vi "VisionExecute.v.vi"   [LabVIEW 2023]
uses:
  <vilib>/Rock Robotics/WPI/ThirdParty/PhotonVisionLib/Enum/PhotonPoseStrategy_ENUM.ctl
  <vilib>/Rock Robotics/WPI/ThirdParty/JAS_Junk/TrajLib/TypeDef/POSE2D.ctl
  <vilib>/Rock Robotics/WPI/ThirdParty/JAS_Junk/TrajLib/TypeDef/TRANSLATION2D.ctl
  <vilib>/Rock Robotics/WPI/ThirdParty/JAS_Junk/TrajLib/TypeDef/ROTATION2D.ctl
  <vilib>/Rock Robotics/WPI/ThirdParty/JAS_Junk/TrajLib/VI/AprilTagFieldLayout_New2025.vi
  <vilib>/Rock Robotics/WPI/ThirdParty/JAS_Junk/TrajLib/VI/Util_GetTime_U32.vi
  <vilib>/Rock Robotics/WPI/ThirdParty/PhotonVisionLib/SubVI/PhotonPipelineResult_Unpack.vi
  <vilib>/Rock Robotics/WPI/ThirdParty/PhotonVisionLib/SubVI/PhotonPipelineResult_GetTargetCount.vi
  <vilib>/Rock Robotics/WPI/ThirdParty/PhotonVisionLib/SubVI/PhotonPipelineResult_GetMetadata.vi
  <vilib>/Rock Robotics/WPI/ThirdParty/PhotonVisionLib/SubVI/PhotonPipelineMetadata_GetAll.vi
  <vilib>/Rock Robotics/WPI/ThirdParty/JAS_Junk/TrajLib/VI/Transform3d_Equals.vi
  <vilib>/Rock Robotics/WPI/ThirdParty/PhotonVisionLib/SubVI/PhotonPoseEstimator_SetCamera.vi
  <vilib>/Rock Robotics/WPI/ThirdParty/PhotonVisionLib/SubVI/PhotonPoseEstimator_SetPrimaryStategy.vi
  <vilib>/Rock Robotics/WPI/ThirdParty/PhotonVisionLib/SubVI/PhotonPoseEstimator_SetMultiTagFallbackStrategy.vi
  <vilib>/Rock Robotics/WPI/ThirdParty/PhotonVisionLib/SubVI/PhotonPoseEstimator_SetHighestAmbiguity.vi
  <vilib>/Rock Robotics/WPI/ThirdParty/PhotonVisionLib/SubVI/PhotonPoseEstimator_SetRobotToCameraTransform.vi
  <vilib>/Rock Robotics/WPI/ThirdParty/PhotonVisionLib/SubVI/PhotonPoseEstimator_New.vi
  <vilib>/Rock Robotics/WPI/ThirdParty/PhotonVisionLib/SubVI/PhotonPoseEstimator_SetLastPose.vi
  <vilib>/Rock Robotics/WPI/ThirdParty/PhotonVisionLib/SubVI/PhotonPoseEstimator_Update_PipeResult.vi
  <vilib>/Rock Robotics/WPI/ThirdParty/PhotonVisionLib/SubVI/PhotonPoseEstimator_SetReferencePose.vi
  <vilib>/Rock Robotics/WPI/ThirdParty/PhotonVisionLib/SubVI/PhotonEstimatedRobotPose_GetAll.vi
  <vilib>/Rock Robotics/WPI/ThirdParty/JAS_Junk/TrajLib/VI/Pose3d_ToPose2d.vi
  <vilib>/Rock Robotics/WPI/ThirdParty/JAS_Junk/TrajLib/VI/Quaternion_New.vi
  <vilib>/Rock Robotics/WPI/ThirdParty/JAS_Junk/TrajLib/Conv_Deg_Radians.vi
  <vilib>/Rock Robotics/WPI/ThirdParty/JAS_Junk/TrajLib/Translation2d_GetDistance.vi
  <vilib>/Rock Robotics/WPI/ThirdParty/JAS_Junk/TrajLib/Rotation2d_Minus.vi
  <vilib>/Rock Robotics/WPI/ThirdParty/JAS_Junk/TrajLib/Rotation2d_GetRadians.vi
  <vilib>/Rock Robotics/WPI/ThirdParty/JAS_Junk/TrajLib/VI/AprilTagFieldLayout_New.vi
  <vilib>/Rock Robotics/WPI/ThirdParty/JAS_Junk/TrajLib/VI/Pose3d_New_Trans3dRot3d.vi
  <vilib>/Rock Robotics/WPI/ThirdParty/JAS_Junk/TrajLib/VI/Rotation3d_Create_Quaternion.vi
  <vilib>/Rock Robotics/WPI/ThirdParty/JAS_Junk/TrajLib/VI/AprilTag_New.vi
  <vilib>/Rock Robotics/WPI/ThirdParty/JAS_Junk/TrajLib/Timer_New.vi
  <vilib>/Rock Robotics/WPI/ThirdParty/PhotonVisionLib/SubVI/Packet_decode_ByteI8.vi
  <vilib>/Rock Robotics/WPI/ThirdParty/PhotonVisionLib/SubVI/PhotonTrackedTarget_Unpack.vi
  <vilib>/Rock Robotics/WPI/ThirdParty/PhotonVisionLib/SubVI/PhotonMultiTargetPNPResult_unpack.vi
  <vilib>/Rock Robotics/WPI/ThirdParty/PhotonVisionLib/SubVI/PhotonPipelineMetadata_Unpack.vi
  <vilib>/Rock Robotics/WPI/ThirdParty/PhotonVisionLib/SubVI/PhotonPipelineResult_New.vi
  <vilib>/Rock Robotics/WPI/ThirdParty/JAS_Junk/TrajLib/VI/Transform3d_GetTranslation3d.vi
  <vilib>/Rock Robotics/WPI/ThirdParty/JAS_Junk/TrajLib/VI/Transform3d_GetRotation3d.vi
  <vilib>/Rock Robotics/WPI/ThirdParty/JAS_Junk/TrajLib/VI/Rotation3d_Equals.vi
  <vilib>/Rock Robotics/WPI/ThirdParty/JAS_Junk/TrajLib/VI/Translation3d_Equals.vi
  <vilib>/Rock Robotics/WPI/ThirdParty/PhotonVisionLib/SubVI/PhotonTargetModel_New_AprilTag36H11.vi
  <vilib>/Rock Robotics/WPI/ThirdParty/PhotonVisionLib/SubVI/PhotonPoseEstimator_Update_All.vi
  <vilib>/Rock Robotics/WPI/ThirdParty/JAS_Junk/TrajLib/VI/Pose3d_getTranslation3d.vi
  <vilib>/Rock Robotics/WPI/ThirdParty/JAS_Junk/TrajLib/VI/Pose3d_getRotation3d.vi
  <vilib>/Rock Robotics/WPI/ThirdParty/JAS_Junk/TrajLib/VI/Translation3d_ToTranslation2d.vi
  <vilib>/Rock Robotics/WPI/ThirdParty/JAS_Junk/TrajLib/VI/Rotation3d_ToRotation2d.vi
  <vilib>/Rock Robotics/WPI/ThirdParty/JAS_Junk/TrajLib/Pose2d_New_TRRO.vi
  <vilib>/Rock Robotics/WPI/ThirdParty/JAS_Junk/TrajLib/Util_CalcDist.vi
  <vilib>/Rock Robotics/WPI/ThirdParty/JAS_Junk/TrajLib/Rotation2d_UnaryMinus.vi
  <vilib>/Rock Robotics/WPI/ThirdParty/JAS_Junk/TrajLib/Rotation2d_RotateBy.vi
  <vilib>/Rock Robotics/WPI/ThirdParty/JAS_Junk/TrajLib/VI/AprilTag_GetAll.vi
  <vilib>/Rock Robotics/WPI/ThirdParty/JAS_Junk/TrajLib/VI/Quaternion_Normalize.vi
  <vilib>/Rock Robotics/WPI/ThirdParty/PhotonVisionLib/SubVI/Packet_decode_Flt64.vi
  <vilib>/Rock Robotics/WPI/ThirdParty/PhotonVisionLib/SubVI/TargetCorner_New.vi
  <vilib>/Rock Robotics/WPI/ThirdParty/PhotonVisionLib/SubVI/Packet_decode_Int32.vi
  <vilib>/Rock Robotics/WPI/ThirdParty/PhotonVisionLib/SubVI/Packet_decode_Transform3d.vi
  <vilib>/Rock Robotics/WPI/ThirdParty/PhotonVisionLib/SubVI/Packet_decode_Flt32.vi
  <vilib>/Rock Robotics/WPI/ThirdParty/PhotonVisionLib/SubVI/Packet_decode_TargetCornerArray.vi
  <vilib>/Rock Robotics/WPI/ThirdParty/PhotonVisionLib/SubVI/Packet_decode_Boolean.vi
  <vilib>/Rock Robotics/WPI/ThirdParty/PhotonVisionLib/SubVI/PhotonPNPResult_unpack.vi
  <vilib>/Rock Robotics/WPI/ThirdParty/PhotonVisionLib/SubVI/PhotonMultiTargetPNPResult_New.vi
  <vilib>/Rock Robotics/WPI/ThirdParty/PhotonVisionLib/SubVI/Packet_decode_Int16.vi
  <vilib>/Rock Robotics/WPI/ThirdParty/PhotonVisionLib/SubVI/Packet_decode_Int64.vi
  <vilib>/Rock Robotics/WPI/ThirdParty/JAS_Junk/TrajLib/VI/Rotation3d_GetQuaterion.vi
  <vilib>/Rock Robotics/WPI/ThirdParty/JAS_Junk/TrajLib/VI/Quaternion_Equals.vi
  <vilib>/Rock Robotics/WPI/ThirdParty/PhotonVisionLib/SubVI/PhotonTargetModel_New_RectPlanar.vi
  <vilib>/Rock Robotics/WPI/ThirdParty/PhotonVisionLib/SubVI/PhotonPoseEstimator_GetEmptyPose.vi
  <vilib>/Rock Robotics/WPI/ThirdParty/PhotonVisionLib/SubVI/PhotonPoseEstimator_lowestAmbiguityStrategy.vi
  <vilib>/Rock Robotics/WPI/ThirdParty/PhotonVisionLib/SubVI/PhotonPoseEstimator_closestToCameraHeightStrategy.vi
  <vilib>/Rock Robotics/WPI/ThirdParty/PhotonVisionLib/SubVI/PhotonPoseEstimator_closestToReferencePoseStrategy.vi
  <vilib>/Rock Robotics/WPI/ThirdParty/PhotonVisionLib/SubVI/PhotonPoseEstimator_GetReferencePose.vi
  <vilib>/Rock Robotics/WPI/ThirdParty/PhotonVisionLib/SubVI/PhotonPoseEstimator_GetLastPose.vi
  <vilib>/Rock Robotics/WPI/ThirdParty/PhotonVisionLib/SubVI/PhotonPoseEstimator_averageBestTargetsStrategy.vi
  <vilib>/Rock Robotics/WPI/ThirdParty/PhotonVisionLib/SubVI/PhotonPoseEstimator_multiTagOnCoprocStrategy.vi
  <vilib>/Rock Robotics/WPI/ThirdParty/PhotonVisionLib/SubVI/PhotonPipelineResult_GetTimeStampSecs.vi
  <vilib>/Rock Robotics/WPI/ThirdParty/JAS_Junk/TrajLib/Translation2d_Create.vi
  <vilib>/Rock Robotics/WPI/ThirdParty/JAS_Junk/TrajLib/Rotation2d_CreateAngle.vi
  <vilib>/Rock Robotics/WPI/ThirdParty/JAS_Junk/TrajLib/VI/Rotation3d_GetXYZ.vi
  <vilib>/Rock Robotics/WPI/ThirdParty/JAS_Junk/TrajLib/Rotation2d_CreateXY.vi
  <vilib>/Rock Robotics/WPI/ThirdParty/JAS_Junk/TrajLib/VI/Quaternion_New_Default.vi
  <vilib>/Rock Robotics/WPI/ThirdParty/PhotonVisionLib/SubVI/PhotonPNPResult_New.vi
  <vilib>/Rock Robotics/WPI/ThirdParty/JAS_Junk/TrajLib/VI/Quaternion_Get_Vect.vi
  <vilib>/Rock Robotics/WPI/ThirdParty/JAS_Junk/TrajLib/VI/Quaternion_Get_W.vi
  <vilib>/Rock Robotics/WPI/ThirdParty/PhotonVisionLib/SubVI/PhotonTargetModel_New.vi
  <vilib>/Rock Robotics/WPI/ThirdParty/JAS_Junk/TrajLib/VI/Rotation3d_Create_AxisAngle.vi
  <vilib>/Rock Robotics/WPI/ThirdParty/JAS_Junk/TrajLib/VI/Pose3d_New.vi
  <vilib>/Rock Robotics/WPI/ThirdParty/PhotonVisionLib/SubVI/PhotonPipelineResult_HasTargets.vi
  <vilib>/Rock Robotics/WPI/ThirdParty/PhotonVisionLib/SubVI/PhotonPipelineResult_GetTargets.vi
  <vilib>/Rock Robotics/WPI/ThirdParty/PhotonVisionLib/SubVI/PhotonTrackedTarget_GetPoseAmbiguity.vi
  <vilib>/Rock Robotics/WPI/ThirdParty/PhotonVisionLib/SubVI/PhotonTrackedTarget_GetFiducialId.vi
  <vilib>/Rock Robotics/WPI/ThirdParty/PhotonVisionLib/SubVI/PhotonPoseEstimator_GetFieldTags.vi
  <vilib>/Rock Robotics/WPI/ThirdParty/JAS_Junk/TrajLib/VI/AprilTagFieldLayout_GetTagPose.vi
  <vilib>/Rock Robotics/WPI/ThirdParty/JAS_Junk/TrajLib/VI/Pose3d_TransformBy.vi
  <vilib>/Rock Robotics/WPI/ThirdParty/PhotonVisionLib/SubVI/PhotonTrackedTarget_GetBestCameraToTarget.vi
  <vilib>/Rock Robotics/WPI/ThirdParty/JAS_Junk/TrajLib/VI/Transform3d_Inverse.vi
  <vilib>/Rock Robotics/WPI/ThirdParty/PhotonVisionLib/SubVI/PhotonPoseEstimator_GetRobotToCameraTransform.vi
  <vilib>/Rock Robotics/WPI/ThirdParty/PhotonVisionLib/SubVI/PhotonPoseEstimator_GetHighestAmbiguity.vi
  <vilib>/Rock Robotics/WPI/ThirdParty/PhotonVisionLib/SubVI/PhotonEstimatedRobotPose_New.vi
  <vilib>/Rock Robotics/WPI/ThirdParty/PhotonVisionLib/SubVI/PhotonPoseEstimator_closestToCameraHeightStrategy_calc.vi
  <vilib>/Rock Robotics/WPI/ThirdParty/PhotonVisionLib/SubVI/PhotonTrackedTarget_GetAltCameraToTarget.vi
  <vilib>/Rock Robotics/WPI/ThirdParty/PhotonVisionLib/SubVI/PhotonPoseEstimator_closestToReferencePoseStrategy_calc.vi
  <vilib>/Rock Robotics/WPI/ThirdParty/PhotonVisionLib/SubVI/PhotonPoseEstimator_averageBestTargetsStrategy_calc.vi
  <vilib>/Rock Robotics/WPI/ThirdParty/JAS_Junk/TrajLib/VI/Rotation3d_Plus.vi
  <vilib>/Rock Robotics/WPI/ThirdParty/JAS_Junk/TrajLib/VI/Translation3d_Plus.vi
  <vilib>/Rock Robotics/WPI/ThirdParty/JAS_Junk/TrajLib/VI/Translation3d_Times.vi
  <vilib>/Rock Robotics/WPI/ThirdParty/JAS_Junk/TrajLib/VI/Rotation3d_Times.vi
  <vilib>/Rock Robotics/WPI/ThirdParty/JAS_Junk/TrajLib/VI/Rotation3d_Create_Default.vi
  <vilib>/Rock Robotics/WPI/ThirdParty/JAS_Junk/TrajLib/VI/Translation3d_Create_Default.vi
  <vilib>/Rock Robotics/WPI/ThirdParty/JAS_Junk/TrajLib/VI/Pose3d_New_Default.vi
  <vilib>/Rock Robotics/WPI/ThirdParty/JAS_Junk/TrajLib/VI/Pose3d_Plus.vi
  <vilib>/Rock Robotics/WPI/ThirdParty/JAS_Junk/TrajLib/VI/Pose3d_RelativeTo.vi
  <vilib>/Rock Robotics/WPI/ThirdParty/JAS_Junk/TrajLib/VI/AprilTagFieldLayout_GetOriginPosition.vi
  <vilib>/Rock Robotics/WPI/ThirdParty/PhotonVisionLib/SubVI/PhotonPipelineResult_GetMultiTagResult.vi
  <vilib>/Rock Robotics/WPI/ThirdParty/JAS_Junk/TrajLib/VI/Quaternion_Get_All.vi
  <vilib>/Rock Robotics/WPI/ThirdParty/JAS_Junk/TrajLib/VI/Vector_Norm.vi
  <vilib>/Rock Robotics/WPI/ThirdParty/JAS_Junk/TrajLib/VecBuilder_ArrayBy1Fill.vi
  <vilib>/Rock Robotics/WPI/ThirdParty/JAS_Junk/TrajLib/VI/Translation3d_RotateBy.vi
  <vilib>/Rock Robotics/WPI/ThirdParty/JAS_Junk/TrajLib/Transform2d_Create_TransRot.vi
  <vilib>/Rock Robotics/WPI/ThirdParty/JAS_Junk/TrajLib/VI/Rotation3d_UnaryMinus.vi
  <vilib>/Rock Robotics/WPI/ThirdParty/JAS_Junk/TrajLib/VI/Translation3d_UnaryMinus.vi
  <vilib>/Rock Robotics/WPI/ThirdParty/JAS_Junk/TrajLib/VI/Transform3d_GetXYZ.vi
  <vilib>/Rock Robotics/WPI/ThirdParty/JAS_Junk/TrajLib/VI/Pose3d_getXYZ.vi
  <vilib>/Rock Robotics/WPI/ThirdParty/PhotonVisionLib/SubVI/PhotonPoseEstimator_CalcDifference.vi
  <vilib>/Rock Robotics/WPI/ThirdParty/JAS_Junk/TrajLib/VI/Rotation3d_RotateBy.vi
  <vilib>/Rock Robotics/WPI/ThirdParty/JAS_Junk/TrajLib/VI/Translation3d_GetXYZ.vi
  <vilib>/Rock Robotics/WPI/ThirdParty/JAS_Junk/TrajLib/VI/Transform3d_Create_Pose3dPose3d.vi
  <vilib>/Rock Robotics/WPI/ThirdParty/JAS_Junk/TrajLib/MatBuilder_Create.vi
  <vilib>/Rock Robotics/WPI/ThirdParty/JAS_Junk/TrajLib/VI/Quaternion_Times.vi
  <vilib>/Rock Robotics/WPI/ThirdParty/JAS_Junk/TrajLib/VI/Quaternion_Inverse.vi
  <vilib>/Rock Robotics/WPI/ThirdParty/JAS_Junk/TrajLib/VI/Translation3d_GetDistance.vi
  <vilib>/Rock Robotics/WPI/ThirdParty/JAS_Junk/TrajLib/VI/Translation3d_Minus.vi
  <vilib>/Rock Robotics/WPI/ThirdParty/JAS_Junk/TrajLib/VI/Rotation3d_Minus.vi
  Robot Global Data.vi
  VisionGlobal.vi
  <vilib>/Rock Robotics/SystemInterfaces/Utilities/FPGA_UtilitiesRead LocalTime.vi
  <vilib>/Rock Robotics/WPI/ThirdParty/JAS_Junk/TrajLib/VI/Util_GetTime_U64.vi
  <vilib>/Utility/semaphor.llb/Obtain Semaphore Reference.vi
  <vilib>/Rock Robotics/WPI/ThirdParty/JAS_Junk/TrajLib/Timer_Reset.vi
  <vilib>/Rock Robotics/WPI/ThirdParty/JAS_Junk/TrajLib/Timer_Start.vi
  <vilib>/Rock Robotics/WPI/ThirdParty/JAS_Junk/TrajLib/Timer_Stop.vi
  <vilib>/Rock Robotics/WPI/ThirdParty/JAS_Junk/TrajLib/Timer_HasPeriodPassedOnce.vi
  <vilib>/Rock Robotics/Network Tables/NT Read Value.vi
  <vilib>/Rock Robotics/Network Tables/NT Read Raw.vi
  <vilib>/Rock Robotics/WPI/ThirdParty/JAS_Junk/TrajLib/Trajectory_Library.lvlib
  <vilib>/Rock Robotics/WPI/ThirdParty/PhotonVisionLib/PhotonVisionLib.lvlib
types:
  T1 = typedef "PhotonVisionLib.lvlib/PhotonPoseStrategy_ENUM.ctl" = enum16{"LOWEST_AMBIGUITY", "CLOSEST_TO_CAMERA_HEIGHT", "CLOSEST_TO_REFERENCE_POSE", "CLOSEST_TO_LAST_POSE", "AVERAGE_BEST_TARGETS", "MULTI_TAG_PNP_ON_COPROCESSOR", "MULTI_TAG_PNP_ON_RIO"}
  T2 = typedef "Trajectory_Library.lvlib/TRANSLATION3D.ctl" = cluster{"X":dbl, "Y":dbl, "Z":dbl}
  T3 = typedef "Trajectory_Library.lvlib/ROTATION3D.ctl" = cluster{"Q_quaternion":T4}
  T4 = typedef "Trajectory_Library.lvlib/QUATERNION.ctl" = cluster{"R":dbl, "V":dbl[]}
  T5 = typedef "Trajectory_Library.lvlib/TRANSFORM3D.ctl" = cluster{"TRANSLATION3D":T2, "ROTATION3D":T3, "XF":bool}
  T6 = typedef "PhotonVisionLib.lvlib/PhotonPipelineResultType.ctl" = cluster{"Targets":T7[], "PhotonMultiTargetPNPResult":T9, "PhotonPipelineMetadata":T11}
  T7 = typedef "PhotonVisionLib.lvlib/PhotonTrackedTargetType.ctl" = cluster{"Yaw":dbl, "Pitch":dbl, "Area":dbl, "Skew":dbl, "MinAreaRectCorners":T8[], "BestCameraToTarget":T5, "FiducialId":i32, "AltCameraToTarget":T5, "PoseAmbiguity":dbl, "DetectedCorners":T8[], "ObjDetectId":i32, "ObjDetectConf":sgl}
  T8 = typedef "PhotonVisionLib.lvlib/TargetCornerType.ctl" = cluster{"X":dbl, "Y":dbl}
  T9 = typedef "PhotonVisionLib.lvlib/PhotonMultiTargetPNPResultType.ctl" = cluster{"PhotonPNPResult":T10, "FiducialIDsUsed":i16[]}
  T10 = typedef "PhotonVisionLib.lvlib/PhotonPNPResultType.ctl" = cluster{"IsPresent":bool, "bestReprojErr":dbl, "altReprojErr":dbl, "ambiguity":dbl, "Best":T5, "Alt":T5}
  T11 = typedef "PhotonVisionLib.lvlib/PhotonPipelineMetadataType.ctl" = cluster{"CaptureTimestampMicros":i64, "PublishTimestampMicros":i64, "SequenceID":i64, "TimeSinceLastPong":i64}
  T12 = typedef "Trajectory_Library.lvlib/AprilTagFieldLayout.ctl" = cluster{"AprilTagMap":map{i32, T13}, "FieldLength":dbl, "FieldWidth":dbl, "OriginPosition ":T15, "OriginPose3d":T14}
  T13 = typedef "Trajectory_Library.lvlib/AprilTag.ctl" = cluster{"ID":i32, "POSE3D":T14}
  T14 = typedef "Trajectory_Library.lvlib/POSE3D.ctl" = cluster{"Translation3d":T2, "Rotation3d":T3}
  T15 = typedef "Trajectory_Library.lvlib/AprilTagFieldLayoutOrignPosition_ENUM.ctl" = enum16{"kBlueAllianceWallRightSide,", "kRedAllianceWallRightSide,"}
  T16 = typedef "PhotonVisionLib.lvlib/PhotonPoseEstimator_Configuration.ctl" = cluster{"Primary Strategy":T1, "Camera":string, "Initial Pose":T14, "HighestAmbiguity":dbl, "RobotToCamera":T5, "FallBack Strategy":T1, "BaseNTName":string}
  T17 = typedef "Trajectory_Library.lvlib/SWERVE_DRIVE_KINEMATICS.ctl" = cluster{"NumModules":i32, "InverseKinematics":T18, "ForwardKinematics":T18, "Modules":T19[], "PrevCoR":T19, "SavedModuleStates":T20[]}
  T18 = typedef "NI_Matrix.lvlib/RealMatrix.ctl" = dbl[][]
  T19 = typedef "Trajectory_Library.lvlib/TRANSLATION2D.ctl" = cluster{"X":dbl, "Y":dbl}
  T20 = typedef "Trajectory_Library.lvlib/SWERVE_DRIVE_MODULE_STATE.ctl" = cluster{"Speed":dbl, "Angle":T21}
  T21 = typedef "Trajectory_Library.lvlib/ROTATION2D.ctl" = cluster{"VALUE":dbl, "COS":dbl, "SIN":dbl}
  T22 = typedef "Trajectory_Library.lvlib/SWERVE_DRIVE_MODULE_POSITION.ctl" = cluster{"Distance":dbl, "Angle":T21, "P":bool}
  T23 = typedef "Trajectory_Library.lvlib/SWERVE_DRIVE_POSE_EST2_CONFIG.ctl" = cluster{"Wheel_Locations M":T19[], "Odom X std dev M":dbl, "Odom Y std dev M":dbl, "Odom Heading std dev Rad":dbl, "Vision X std dev M":dbl, "Vision Y std dev M":dbl, "Vision Heading std dev Rad":dbl}
  T24 = typedef "Trajectory_Library.lvlib/POSE2D.ctl" = cluster{"TRANSLATION":T19, "ROTATION":T21}
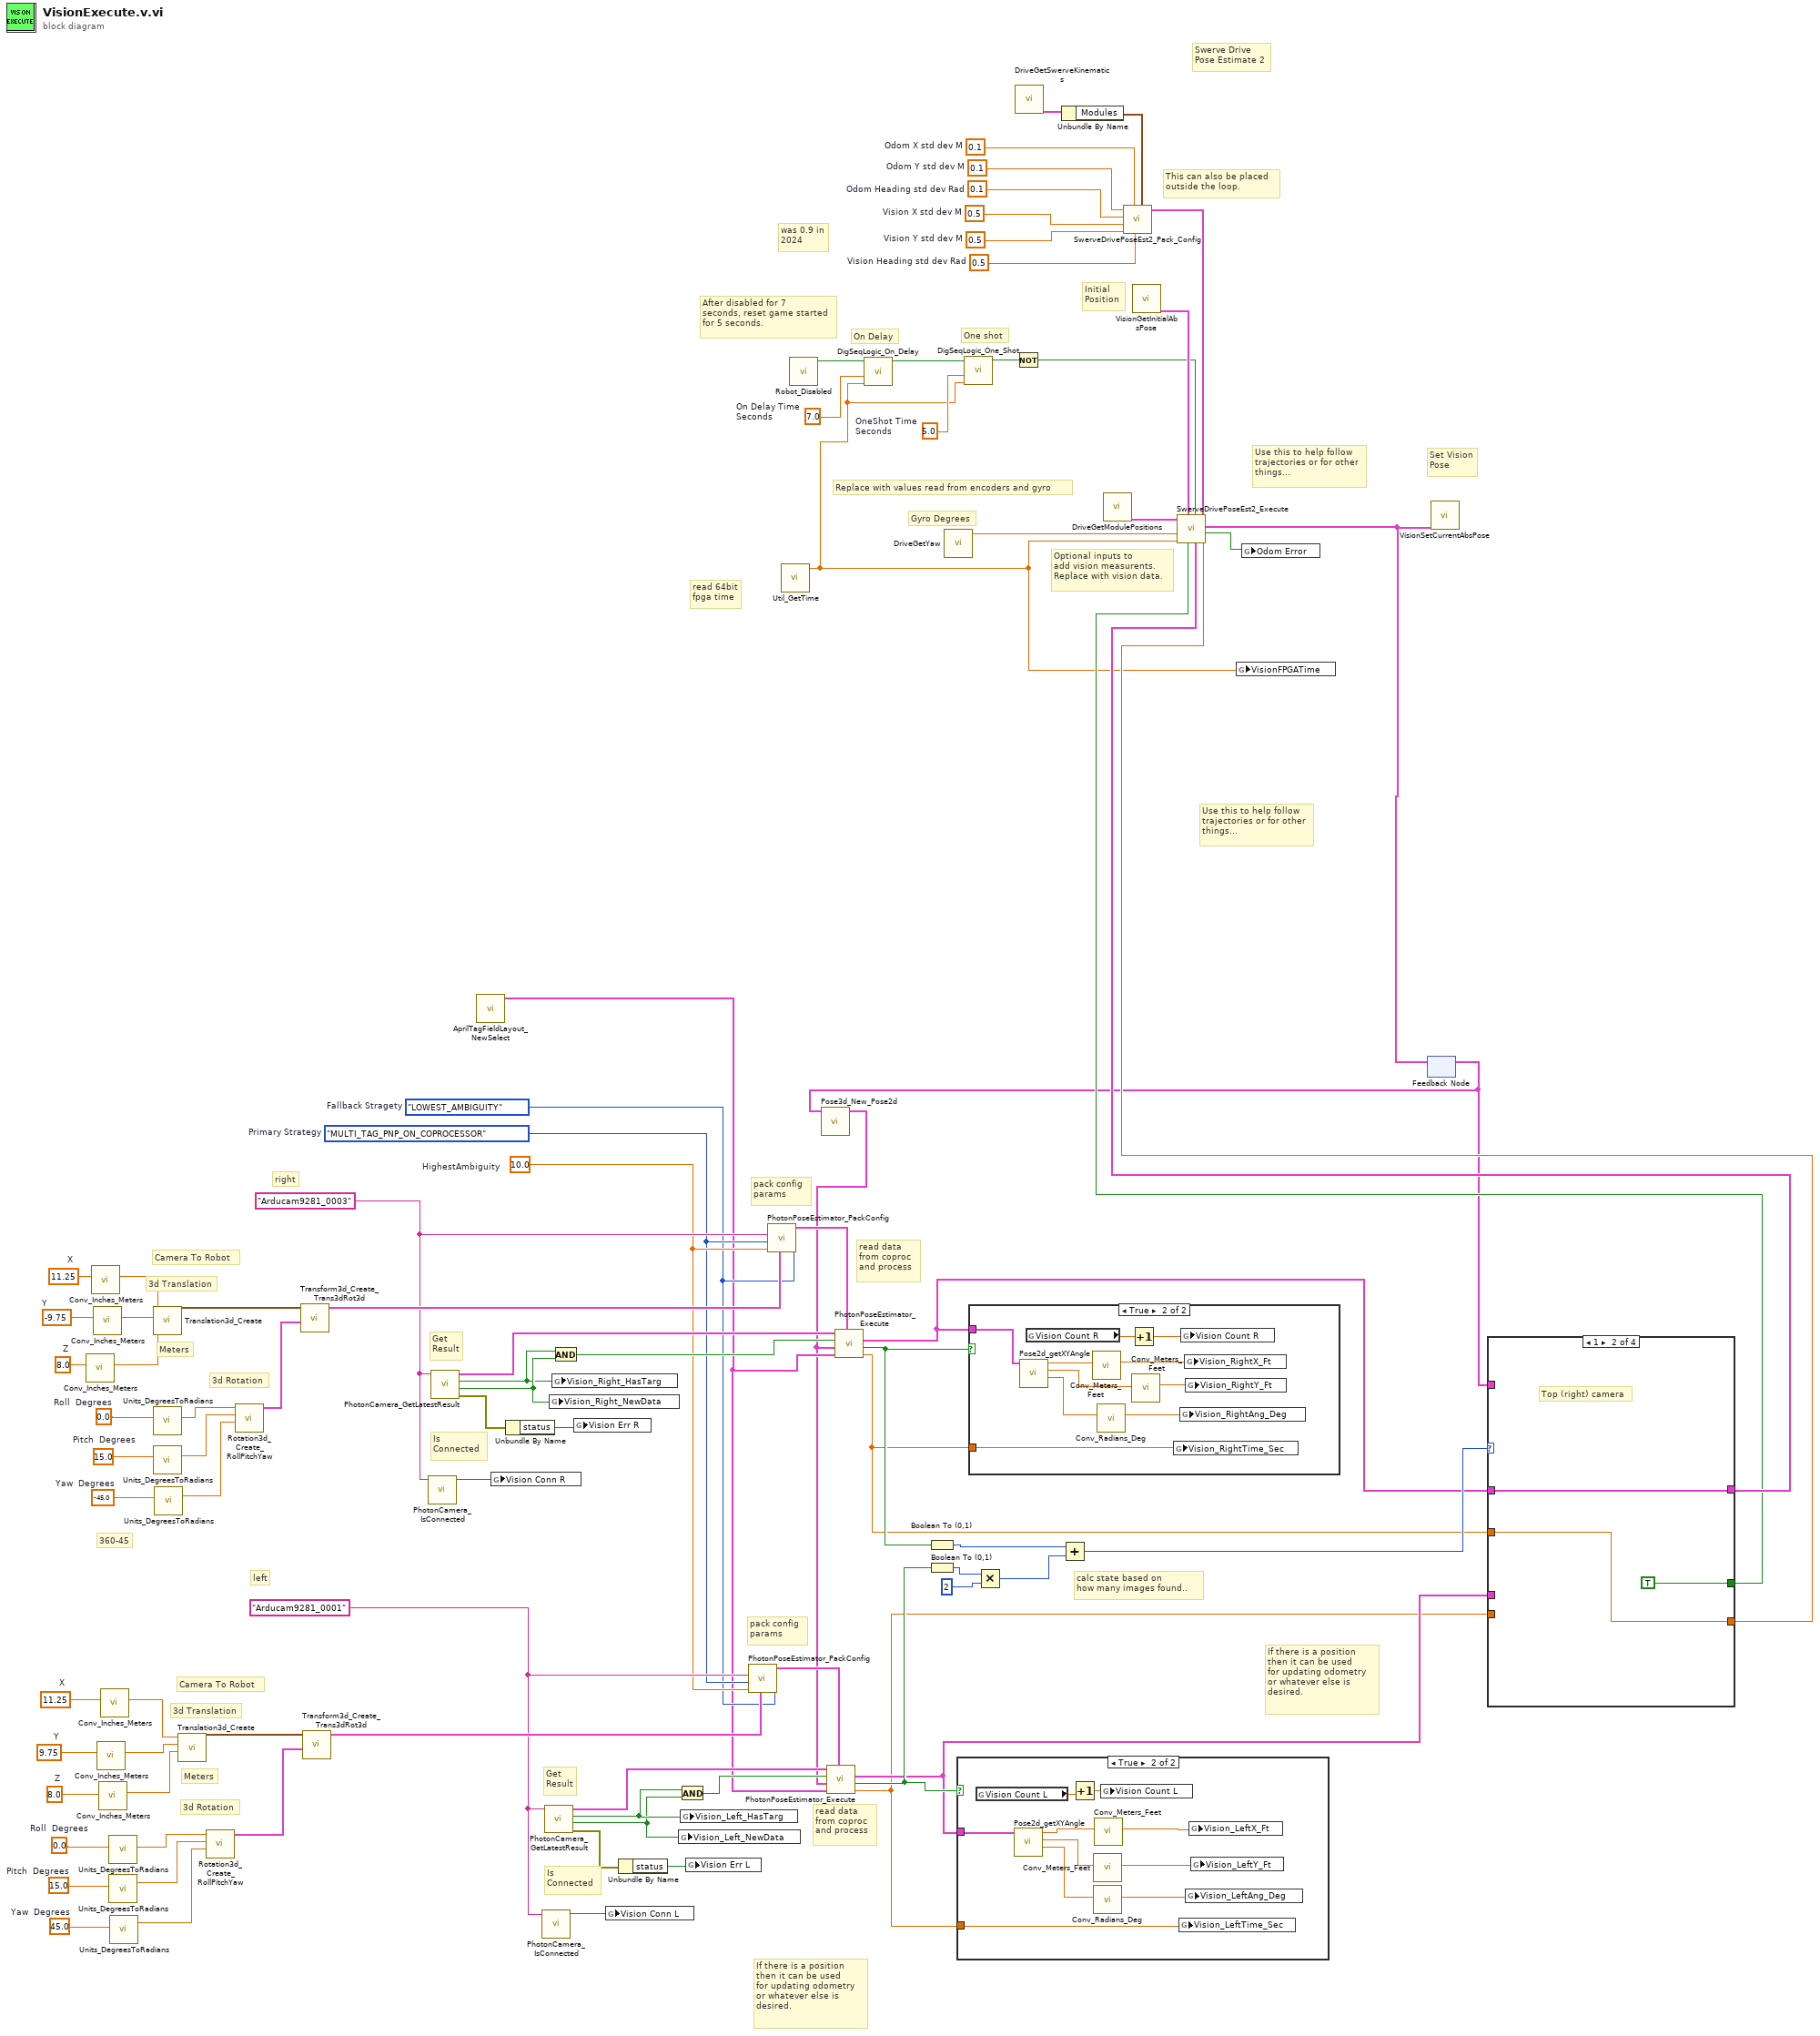
[diagram p0: block diagram]
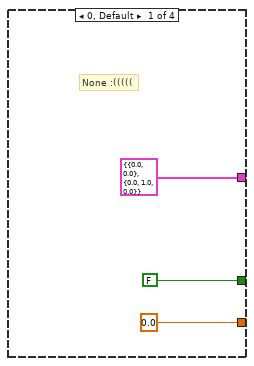
[diagram p2: hidden frame]
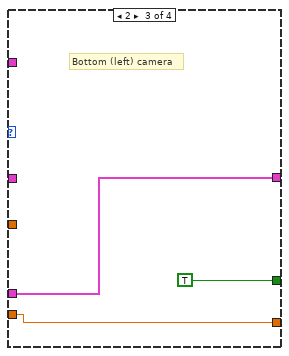
[diagram p3: hidden frame]
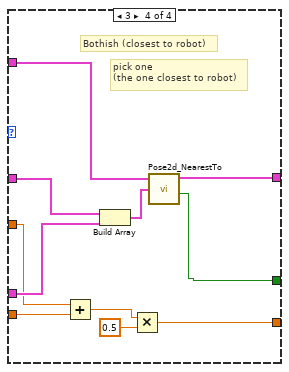
[diagram p4: hidden frame]
diagram:
  w11 = 5.0  # OneShot Time Seconds
  w13 = 7.0  # On Delay Time Seconds
  w21 = PhotonPoseStrategy_ENUM."LOWEST_AMBIGUITY"  # Fallback Stragety
  w31 = 0.1  # Odom Y std dev M
  w32 = 0.1  # Odom Heading std dev Rad
  w33 = 0.5  # Vision X std dev M
  w34 = 0.5  # Vision Y std dev M
  w35 = 0.1  # Odom X std dev M
  w36 = 0.5  # Vision Heading std dev Rad
  w68 = 0.0  # Roll  Degrees
  w67 = 15.0  # Pitch  Degrees
  w66 = 45.0  # Yaw  Degrees
  w53 = 8.0  # Z
  w57 = 11.25  # X
  w55 = 9.75  # Y
  w62 = "Arducam9281_0001" ("CameraName")
  w84 = 0.0  # Roll  Degrees
  w83 = 15.0  # Pitch  Degrees
  w82 = -45.0  # Yaw  Degrees
  w47 = 8.0  # Z
  w51 = 11.25  # X
  w49 = -9.75  # Y
  w45 = 10.0  # HighestAmbiguity
  w44 = PhotonPoseStrategy_ENUM."MULTI_TAG_PNP_ON_COPROCESSOR"  # Primary Strategy
  w78 = "Arducam9281_0003" ("CameraName")
  # "Set Vision\nPose"
  # "After disabled for 7\nseconds, reset game started\nfor 5 seconds."
  # "One shot"
  # "On Delay"
  # "360-45"
  # "was 0.9 in\n2024"
  # "calc state based on\nhow many images found.."
  # "read data\nfrom coproc\nand process"
  # "read data\nfrom coproc\nand process"
  # "pack config\nparams"
  # "pack config\nparams"
  # "Initial\nPosition"
  # "Optional inputs to\nadd vision measurents.\nReplace with vision data."
  # "Replace with values read from encoders and gyro"
  # "read 64bit\nfpga time"
  # "This can also be placed \noutside the loop."
  # "Use this to help follow\ntrajectories or for other\nthings..."
  # "Swerve Drive \nPose Estimate 2"
  # "Use this to help follow\ntrajectories or for other\nthings..."
  # "right"
  # "left"
  # "If there is a position\nthen it can be used\nfor updating odometry\nor whatever else is \ndesired."
  # "Meters"
  # "Camera To Robot"
  # "3d Rotation"
  # "3d Translation"
  # "Is\nConnected"
  # "Get\nResult"
  # "If there is a position\nthen it can be used\nfor updating odometry\nor whatever else is \ndesired."
  # "Meters"
  # "Camera To Robot"
  # "3d Rotation"
  # "3d Translation"
  # "Is\nConnected"
  # "Get\nResult"
  # "Gyro Degrees"
  n1 = call <vilib>:"Conv_Inches_Meters.vi"("INCH"=w47) -> ("Meters"=w46:dbl)  [unwired: 10 in]
  n2 = call <vilib>:"Conv_Inches_Meters.vi"("INCH"=w51) -> ("Meters"=w50:dbl)  [unwired: 10 in]
  n3 = call <vilib>:"Conv_Inches_Meters.vi"("INCH"=w49) -> ("Meters"=w48:dbl)  [unwired: 10 in]
  n4 = call <vilib>:"Conv_Inches_Meters.vi"("INCH"=w55) -> ("Meters"=w54:dbl)  [unwired: 10 in]
  n5 = call <vilib>:"Conv_Inches_Meters.vi"("INCH"=w53) -> ("Meters"=w52:dbl)  [unwired: 10 in]
  n6 = call <vilib>:"Conv_Inches_Meters.vi"("INCH"=w57) -> ("Meters"=w56:dbl)  [unwired: 10 in]
  n7 = call <vilib>:"Units_DegreesToRadians.vi"("Degrees"=w68) -> ("Radians"=w65:dbl)  [unwired: 10 in]
  n8 = call <vilib>:"Units_DegreesToRadians.vi"("Degrees"=w67) -> ("Radians"=w64:dbl)  [unwired: 10 in]
  n9 = call <vilib>:"Units_DegreesToRadians.vi"("Degrees"=w66) -> ("Radians"=w63:dbl)  [unwired: 10 in]
  n10 = call <vilib>:"Translation3d_Create.vi"("Z"=w46, "Y"=w48, "X"=w50) -> ("TRANSLATION3D"=w85:T2)  [unwired: 8 in]
  n11 = call <vilib>:"Units_DegreesToRadians.vi"("Degrees"=w84) -> ("Radians"=w81:dbl)  [unwired: 10 in]
  n12 = call <vilib>:"Units_DegreesToRadians.vi"("Degrees"=w83) -> ("Radians"=w80:dbl)  [unwired: 10 in]
  n13 = call <vilib>:"Units_DegreesToRadians.vi"("Degrees"=w82) -> ("Radians"=w79:dbl)  [unwired: 10 in]
  n14 = call <vilib>:"Translation3d_Create.vi"("Z"=w52, "Y"=w54, "X"=w56) -> ("TRANSLATION3D"=w69:T2)  [unwired: 8 in]
  n15 = call <vilib>:"Rotation3d_Create_RollPitchYaw.vi"("Yaw"=w63, "Pitch"=w64, "Roll"=w65) -> ("Rotation3d"=w70:T3)  [unwired: 8 in]
  n16 = call <vilib>:"Rotation3d_Create_RollPitchYaw.vi"("Yaw"=w79, "Pitch"=w80, "Roll"=w81) -> ("Rotation3d"=w86:T3)  [unwired: 8 in]
  n17 = call <vilib>:"Transform3d_Create_Trans3dRot3d.vi"("Rotation3d"=w86, "Translation3d"=w85) -> ("Transform3d"=w87:T5)  [unwired: 9 in]
  n18 = call <vilib>:"Transform3d_Create_Trans3dRot3d.vi"("Rotation3d"=w70, "Translation3d"=w69) -> ("Transform3d"=w71:T5)  [unwired: 9 in]
  n19 = call <vilib>:"PhotonCamera_IsConnected.vi"("CameraName"=w78) -> ("IsConnected"=w76:bool)  [unwired: 9 in, 1 out]
  n20 = call <vilib>:"PhotonCamera_GetLatestResult.vi"("CameraName"=w78) -> ("error out"=w75:errorcluster, "New Data"=w4:bool, "HasTargets"=w3:bool, "PipelineResult"=w88:T6)  [unwired: 6 in, 1 out]
  n21 = call-poly <vilib>:"AprilTagFieldLayout_NewSelect.vi"() -> ("AprilTagFieldLayout"=w14:T12)  [unwired: 11 in]
  n22 = global write "VisionGlobal.vi" "Vision Conn R"(w76) -> ()
  n23 = Unbundle By Name(w75) -> ("status"=w74:bool)
  n24 = call <vilib>:"PhotonCamera_IsConnected.vi"("CameraName"=w62) -> ("IsConnected"=w60:bool)  [unwired: 9 in, 1 out]
  n25 = call <vilib>:"PhotonCamera_GetLatestResult.vi"("CameraName"=w62) -> ("error out"=w59:errorcluster, "New Data"=w1:bool, "HasTargets"=w2:bool, "PipelineResult"=w72:T6)  [unwired: 6 in, 1 out]
  n26 = global write "VisionGlobal.vi" "Vision_Right_NewData"(w4) -> ()
  n27 = And(x=w3, y=w4) -> (x .and. y?=w89:bool)
  n28 = global write "VisionGlobal.vi" "Vision_Right_HasTarg"(w3) -> ()
  n29 = global write "VisionGlobal.vi" "Vision Err R"(w74) -> ()
  n30 = global write "VisionGlobal.vi" "Vision Conn L"(w60) -> ()
  n31 = Unbundle By Name(w59) -> ("status"=w58:bool)
  n32 = And(x=w2, y=w1) -> (x .and. y?=w73:bool)
  n33 = global write "VisionGlobal.vi" "Vision_Left_NewData"(w1) -> ()
  n34 = global write "VisionGlobal.vi" "Vision_Left_HasTarg"(w2) -> ()
  n35 = global write "VisionGlobal.vi" "Vision Err L"(w58) -> ()
  n36 = call <vilib>:"PhotonPoseEstimator_PackConfig.vi"("FallBack Strategy"=w21, "RobotToCamera"=w71, "HighestAmbiguity"=w45, "PirmaryStrategy"=w44, "Camera"=w62) -> ("PoseEstimator_Configuration"=w61:T16)  [unwired: 6 in]
  n37 = call <vilib>:"PhotonPoseEstimator_PackConfig.vi"("FallBack Strategy"=w21, "RobotToCamera"=w87, "HighestAmbiguity"=w45, "PirmaryStrategy"=w44, "Camera"=w78) -> ("PoseEstimator_Configuration"=w77:T16)  [unwired: 6 in]
  n38 = call <vilib>:"Util_GetTime.vi"() -> ("FPGA_Time_Seconds"=w7:dbl)  [unwired: 9 in, 2 out]
  n39 = call "Robot_Disabled.vi"() -> ("Robot Disabled"=w12:bool)  [unwired: 11 in]
  n40 = call <vilib>:"DigSeqLogic_On_Delay.vi"("Time"=w7, "Delay"=w13, "Input"=w12) -> ("Output"=w10:bool)  [unwired: 7 in, 1 out]
  n41 = call "DriveGetYaw.vi"() -> ("Yaw"=w26:dbl)  [unwired: 11 in]
  n42 = call <vilib>:"DigSeqLogic_One_Shot.vi"("Time"=w7, "OneShot"=w11, "Input"=w10) -> ("Output"=w9:bool)  [unwired: 7 in, 1 out]
  n43 = Not(x=w9) -> (.not. x?=w8:bool)
  n44 = call "DriveGetSwerveKinematics.vi"() -> ("SWERVE_DRIVE_KINEMATICS"=w23:T17)  [unwired: 11 in]
  n45 = Unbundle By Name(w23) -> ("Modules"=w22:T19[])
  n46 = call "DriveGetModulePositions.vi"() -> ("Swerve_Drive_Modual_Positions"=w27:T22[])  [unwired: 11 in]
  n47 = call <vilib>:"SwerveDrivePoseEst2_Pack_Config.vi"("Wheel_Locations M"=w22, "Vision Heading std dev Rad"=w36, "Odom X std dev M"=w35, "Vision Y std dev M"=w34, "Vision X std dev M"=w33, "Odom Heading std dev Rad"=w32, "Odom Y std dev M"=w31) -> ("SwervePoseEst2Config"=w30:T23)  [unwired: 4 in]
  n48 = call "VisionGetInitialAbsPose.vi"() -> ("InitialABSPose"=w15:T24)  [unwired: 10 in]
  n49 = global write "VisionGlobal.vi" "VisionFPGATime"(w7) -> ()
  n50 = feedback #1() -> (w6:T24)  [unwired: 1 in]
  n51 = call <vilib>:"Pose3d_New_Pose2d.vi"("in POSE2D"=w6) -> ("out Pose3d"=w5:T14)  [unwired: 10 in]
  n52 = call <vilib>:"PhotonPoseEstimator_Execute.vi"("Configuration"=w61, "AprilTagFieldLayout"=w14, "ReferencePose"=w5, "PIpeline Has \nNew Results"=w73, "PipelineResult"=w72) -> ("TimeStamp_Seconds"=w18:dbl, "New Pose Found"=w42:bool, "EstimatedPose2d"=w20:T24)  [unwired: 4 out]
  n53 = call <vilib>:"PhotonPoseEstimator_Execute.vi"("Configuration"=w77, "AprilTagFieldLayout"=w14, "ReferencePose"=w5, "PIpeline Has \nNew Results"=w89, "PipelineResult"=w88) -> ("TimeStamp_Seconds"=w17:dbl, "New Pose Found"=w43:bool, "EstimatedPose2d"=w19:T24)  [unwired: 4 out]
  n54 = Boolean To (0,1)(Boolean=w43) -> (0, 1=w38:i16)
  n55 = Boolean To (0,1)(Boolean=w42) -> (0, 1=w41:i16)
  n56 = case shown="True" w42 {
    tunnel: w20 -> [_ w97]
    tunnel: w18 -> [_ w90]
    frame False {
    }
    frame True {
      n57 = global read "VisionGlobal.vi" "Vision Count L"() -> (w98:dbl)
      n58 = call <vilib>:"Pose2d_getXYAngle.vi"("in POSE"=w97) -> ("Angle"=w94:dbl, "Y"=w95:dbl, "X"=w96:dbl)  [unwired: 8 in]
      n59 = Increment(x=w98) -> (x+1=w99:dbl)
      n60 = call <vilib>:"Conv_Meters_Feet.vi"("Meters"=w95) -> ("Feet"=w92:dbl)  [unwired: 10 in]
      n61 = call <vilib>:"Conv_Radians_Deg.vi"("Radians"=w94) -> ("Degrees"=w91:dbl)  [unwired: 10 in]
      n62 = call <vilib>:"Conv_Meters_Feet.vi"("Meters"=w96) -> ("Feet"=w93:dbl)  [unwired: 10 in]
      n63 = global write "VisionGlobal.vi" "Vision Count L"(w99) -> ()
      n64 = global write "VisionGlobal.vi" "Vision_LeftTime_Sec"(w90) -> ()
      n65 = global write "VisionGlobal.vi" "Vision_LeftAng_Deg"(w91) -> ()
      n66 = global write "VisionGlobal.vi" "Vision_LeftX_Ft"(w93) -> ()
      n67 = global write "VisionGlobal.vi" "Vision_LeftY_Ft"(w92) -> ()
    }
  }
  n68 = case shown="True" w43 {
    tunnel: w19 -> [_ w107]
    tunnel: w17 -> [_ w100]
    frame False {
    }
    frame True {
      n69 = call <vilib>:"Pose2d_getXYAngle.vi"("in POSE"=w107) -> ("Angle"=w104:dbl, "Y"=w105:dbl, "X"=w106:dbl)  [unwired: 8 in]
      n70 = global read "VisionGlobal.vi" "Vision Count R"() -> (w108:dbl)
      n71 = call <vilib>:"Conv_Meters_Feet.vi"("Meters"=w106) -> ("Feet"=w103:dbl)  [unwired: 10 in]
      n72 = call <vilib>:"Conv_Radians_Deg.vi"("Radians"=w104) -> ("Degrees"=w101:dbl)  [unwired: 10 in]
      n73 = Increment(x=w108) -> (x+1=w109:dbl)
      n74 = call <vilib>:"Conv_Meters_Feet.vi"("Meters"=w105) -> ("Feet"=w102:dbl)  [unwired: 10 in]
      n75 = global write "VisionGlobal.vi" "Vision_RightTime_Sec"(w100) -> ()
      n76 = global write "VisionGlobal.vi" "Vision_RightAng_Deg"(w101) -> ()
      n77 = global write "VisionGlobal.vi" "Vision Count R"(w109) -> ()
      n78 = global write "VisionGlobal.vi" "Vision_RightX_Ft"(w103) -> ()
      n79 = global write "VisionGlobal.vi" "Vision_RightY_Ft"(w102) -> ()
    }
  }
  n80 = Multiply(x=w41, y=i16 2) -> (x*y=w39:i16)
  n81 = Add(x=w38, y=w39) -> (x+y=w37:i16)
  n82 = case shown="1" w37 {
    tunnel: w19 -> [_ w114 _ w127]
    tunnel: w20 -> [_ _ w117 w126]
    tunnel: w6 -> [_ _ _ w128]
    tunnel: [FALSE ("Found") TRUE ("Found") TRUE ("Found") w124] -> w16
    tunnel: w17 -> [_ w115 _ w123]
    tunnel: w18 -> [_ _ w118 w122]
    tunnel: [T24 {"TRANSLATION"={"X"=0.0, "Y"=0.0}, "ROTATION"={"VALUE"=0.0, "COS"=1.0, "SIN"=0.0}} ("Nearest Pose") w114 w117 w125] -> w25
    tunnel: [0.0 w115 w118 w119] -> w24
    frame 0, Default {
      # "None :((((("
    }
    frame 1 {
      # "Top (right) camera"
    }
    frame 2 {
      # "Bottom (left) camera"
    }
    frame 3 {
      # "pick one \n(the one closest to robot)"
      # "Bothish (closest to robot)"
      n83 = Add(x=w123, y=w122) -> (x+y=w121:dbl)
      n84 = Build Array(w127, w126) -> (w129:T24[])
      n85 = Multiply(x=w121, y=0.5) -> (x*y=w119:dbl)
      n86 = call <vilib>:"Pose2d_NearestTo.vi"("other POSE"=w129, "in POSE"=w128) -> ("Found"=w124:bool, "Nearest Pose"=w125:T24)  [unwired: 8 in]
    }
  }
  n87 = call <vilib>:"SwerveDrivePoseEst2_Execute.vi"("Vision TImeStamp_Seconds"=w24, "SwervePoseEst2Config"=w30, "visionRobotPose"=w25, "Game Started"=w8, "Add Vision Meas"=w16, "InitialPose"=w15, "Pass Through Time"=w7, "Gyro Degrees"=w26, "Module Positions"=w27) -> ("Error"=w28:bool, "Estimated Pose"=w29:T24)  [unwired: 1 in]
  n88 = global write "VisionGlobal.vi" "Odom Error"(w28) -> ()
  n89 = feedback-in #1(w29) -> ()
  n90 = call "VisionSetCurrentAbsPose.vi"("Current ABS Pose"=w29) -> ()  [unwired: 11 in]
